vi "Arrange VIWin - Get FP Objects Arrangement Info.vi"(11 "error in":errorcluster) -> (4 "FP objects arrangement info":T1, 15 "error out":errorcluster)   [LabVIEW 2015, in "Arrange VI Window.lvlib"]
uses:
  Arrange VI Window.lvlib
  Arrange VIWin - FP Objects Arrangement Info.ctl
  <resource>/dialog/lvconfig.llb/LV Config Read Numeric (I32).vi
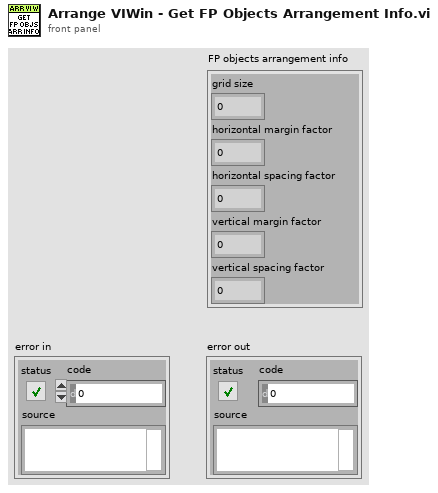
[diagram p1: front panel]
types:
  T1 = typedef "Arrange VI Window.lvlib/Arrange VIWin - FP Objects Arrangement Info.ctl" = cluster{"grid size":i32, "horizontal margin factor":i32, "horizontal spacing factor":i32, "vertical margin factor":i32, "vertical spacing factor":i32}
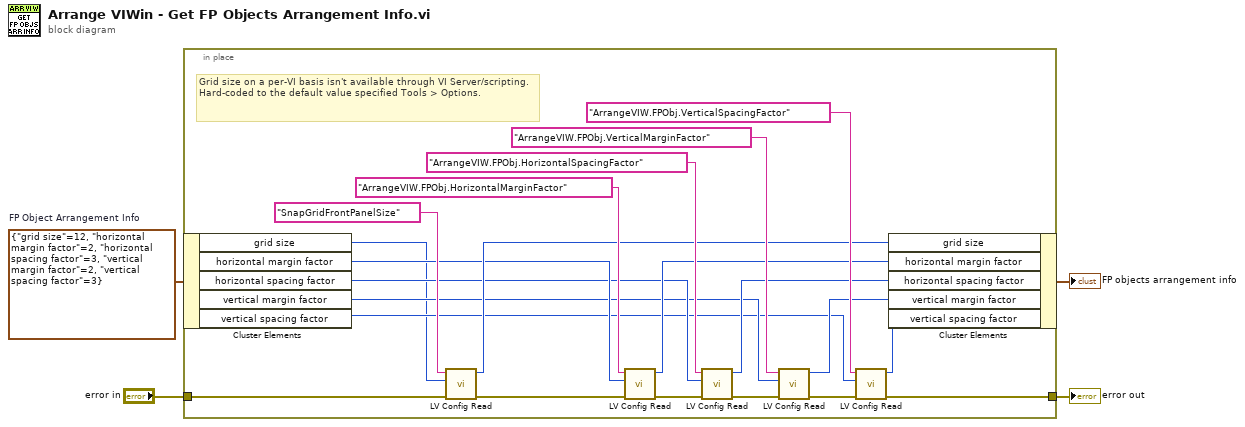
[diagram p0: block diagram]
diagram:
  w2 = T1 {"grid size"=12, "horizontal margin factor"=2, "horizontal spacing factor"=3, "vertical margin factor"=2, "vertical spacing factor"=3}  # FP Object Arrangement Info
  n1 = in-place {
    in-place-border: "error in" -> [w15]
    in-place-border: [w17] -> w3
    # "Grid size on a per-VI basis isn't available through VI Server/scripting.\nHard-coded to the default value specified Tools > Options."
    n2 = in-place-cluster #1(w2) -> ("grid size"=w5:i32, "horizontal margin factor"=w9:i32, "horizontal spacing factor"=w8:i32, "vertical margin factor"=w7:i32, "vertical spacing factor"=w6:i32)
    n3 = call-poly <resource>:"LV Config Read.vi"("error in"=w15, "default value"=w5, "key"="SnapGridFrontPanelSize") -> ("error out"=w16:errorcluster, "value"=w14:i32)  [unwired: 2 in, 1 out]
    n4 = call-poly <resource>:"LV Config Read.vi"("error in"=w16, "default value"=w9, "key"="ArrangeVIW.FPObj.HorizontalMarginFactor") -> ("error out"=w20:errorcluster, "value"=w13:i32)  [unwired: 2 in, 1 out]
    n5 = call-poly <resource>:"LV Config Read.vi"("error in"=w20, "default value"=w8, "key"="ArrangeVIW.FPObj.HorizontalSpacingFactor") -> ("error out"=w19:errorcluster, "value"=w12:i32)  [unwired: 2 in, 1 out]
    n6 = call-poly <resource>:"LV Config Read.vi"("error in"=w19, "default value"=w7, "key"="ArrangeVIW.FPObj.VerticalMarginFactor") -> ("error out"=w18:errorcluster, "value"=w11:i32)  [unwired: 2 in, 1 out]
    n7 = call-poly <resource>:"LV Config Read.vi"("error in"=w18, "default value"=w6, "key"="ArrangeVIW.FPObj.VerticalSpacingFactor") -> ("error out"=w17:errorcluster, "value"=w10:i32)  [unwired: 2 in, 1 out]
    n8 = in-place-cluster #1("grid size"=w14, "horizontal margin factor"=w13, "horizontal spacing factor"=w12, "vertical margin factor"=w11, "vertical spacing factor"=w10) -> (→"FP objects arrangement info":T1)
  }
  "error out" <- w3
